vi "test.MemoryAndSafety.vi"(8 "error in":errorcluster, 10 "Data":variant, 11 "Command":string) -> (0 "error out":errorcluster, 3 "Return Data":variant)   [LabVIEW 2014]
uses:
  Private/Class/meth.Constructor.vi
  Private/Class/meth.Destructor.vi
  GLue.lvlib
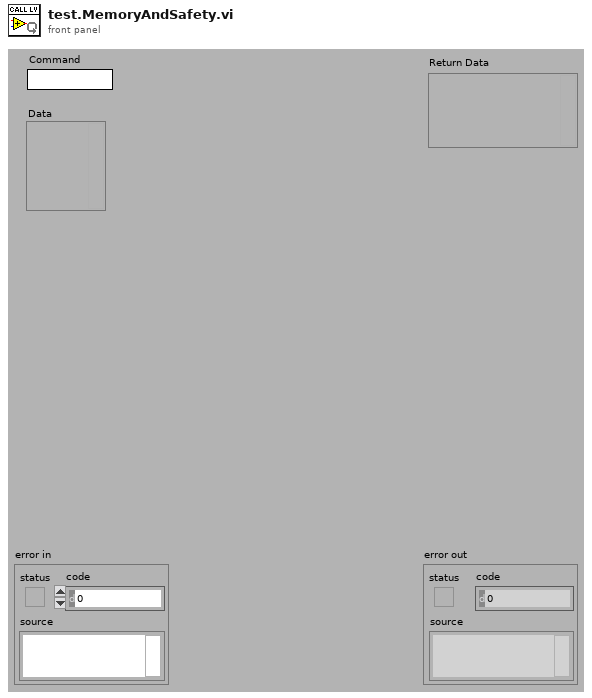
[diagram p1: front panel]
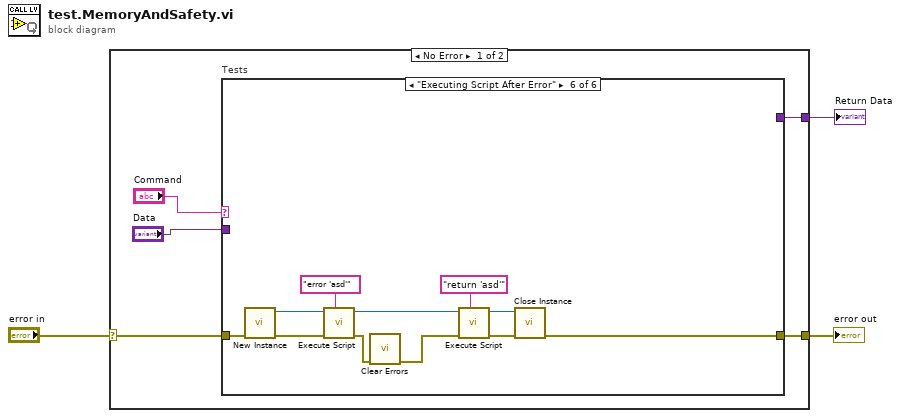
[diagram p0: block diagram]
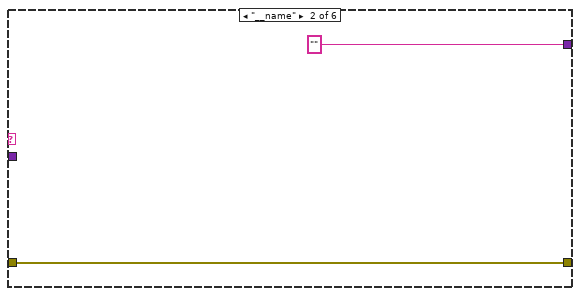
[diagram p3: hidden frame]
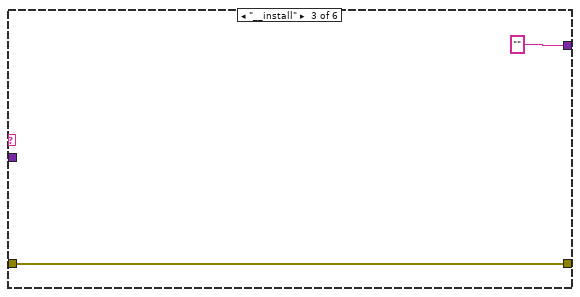
[diagram p4: hidden frame]
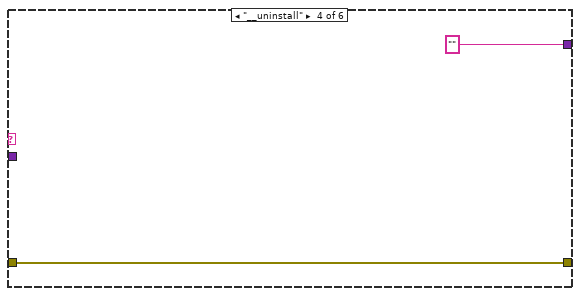
[diagram p5: hidden frame]
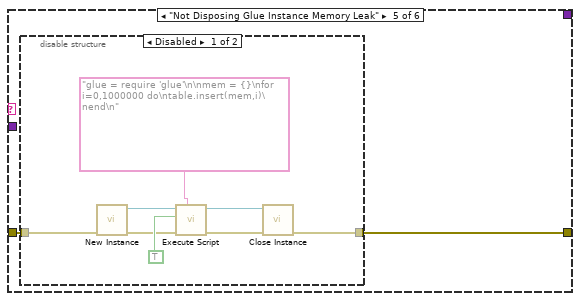
[diagram p6: hidden frame]
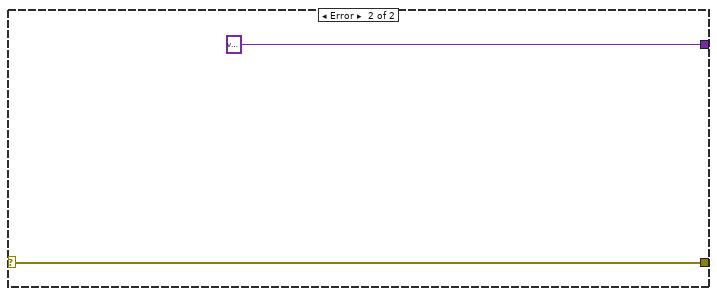
[diagram p8: hidden frame]
diagram:
  n1 = case shown="No Error" "error in" {
    selector: "error in" -> [w8 w39]
    tunnel: [w6 w39] -> w2
    tunnel: [w7 variant ("User Data")] -> w1
    frame No Error {
      n2 = case "Tests" shown="\"Executing Script After Error\"" "Command" {
        tunnel: w8 -> [w10 w11 w13 w15 w18 w35]
        tunnel: "Data" -> [w9 _ _ _ _ _]
        tunnel: [w9 "" "" "" _ _] -> w7
        tunnel: [w10 w11 w13 w15 w17 w28] -> w6
        frame Default {
        }
        frame "__name" {
        }
        frame "__install" {
        }
        frame "__uninstall" {
        }
        frame "Not Disposing Glue Instance Memory Leak" {
          n3 = disable-structure shown="Disabled" {
            disable-tunnel: w18 -> [w23 _]
            disable-tunnel: [w20 _] -> w17
            frame Disabled {
              n4 = call "New Instance.vi"("error in"=w23) -> ("error out"=w24:errorcluster, "GLue out"=w25:refnum<class "class.GLue.lvclass">)  [unwired: 9 in]
              n5 = call "Execute Script.vi"("Script"="glue = require 'glue'\n\nmem = {}\nfor i=0,1000000 do\ntable.insert(mem,i)\nend\n", "error in"=w24, "Argument Data"=TRUE, "GLue in"=w25) -> ("error out"=w21:errorcluster, "GLue out"=w19:refnum<class "class.GLue.lvclass">)  [unwired: 5 in, 1 out]
              n6 = call "Close Instance.vi"("error in"=w21, "GLue in"=w19) -> ("error out"=w20:errorcluster)  [unwired: 9 in]
            }
            frame Enabled {
            }
          }
        }
        frame "Executing Script After Error" {
          n7 = call "New Instance.vi"("error in"=w35) -> ("error out"=w36:errorcluster, "GLue out"=w37:refnum<class "class.GLue.lvclass">)  [unwired: 9 in]
          n8 = call "Execute Script.vi"("Script"="error 'asd'", "error in"=w36, "GLue in"=w37) -> ("error out"=w33:errorcluster, "GLue out"=w29:refnum<class "class.GLue.lvclass">)  [unwired: 6 in, 1 out]
          n9 = call <vilib>:"Clear Errors.vi"("error in (no error)"=w33) -> ("error out"=w30:errorcluster)  [unwired: 5 in, 1 out]
          n10 = call "Execute Script.vi"("Script"="return 'asd'", "error in"=w30, "GLue in"=w29) -> ("error out"=w32:errorcluster, "GLue out"=w31:refnum<class "class.GLue.lvclass">)  [unwired: 6 in, 1 out]
          n11 = call "Close Instance.vi"("error in"=w32, "GLue in"=w31) -> ("error out"=w28:errorcluster)  [unwired: 9 in]
        }
      }
    }
    frame Error {
    }
  }
  "Return Data" <- w1
  "error out" <- w2
